vi "Burst String to Lines.vi"(11 "read buffer":string) -> (3 "lines":string[](array[string]))   [LabVIEW 2013, in "GOLPI library.lvlib"]
uses:
  GOLPI library.lvlib
  <vilib>/Utility/error.llb/whitespace.ctl
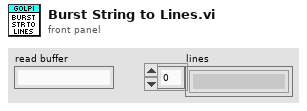
[diagram p1: front panel]
types:
  T1 = typedef "whitespace.ctl" = u16
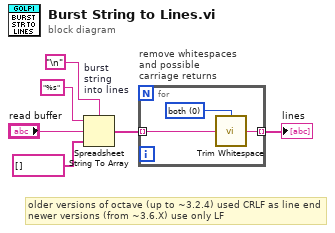
[diagram p0: block diagram]
diagram:
  # "older versions of octave (up to ~3.2.4) used CRLF as line end\nnewer versions (from ~3.6.X) use only LF"
  n1 = Spreadsheet String To Array "burst\nstring\ninto lines"(delimiter (Tab)="\n", format string="%s", spreadsheet string="read buffer", array type (2D Dbl)=string[] []) -> (array=w2:string[])
  n2 = for "remove whitespaces\nand possible\ncarriage returns" {
    tunnel: w2 -> [w9] mode=indexing
    tunnel: [w8] -> w1 mode=indexing
    w7 = T1 0 items=["both", "start of string", "end of string"] ("location (both)")
    n3 = call <vilib>:"Trim Whitespace.vi"("string"=w9, "location (both)"=w7) -> ("trimmed string"=w8:string)
  }
  "lines" <- w1
